vi "get_paths.vi"(8 "error in (no error)":errorcluster, 10 "force file name":string, 11 "GenericComponent in":refnum<class "GenericComponent.lvclass">) -> (0 "error out":errorcluster, 1 "settings paths":T3, 2 "configuration paths":T2, 3 "GenericComponent out":refnum<class "GenericComponent.lvclass">, 5 "component paths":T1)   [LabVIEW 2017, in "GenericComponent.lvclass"]
uses:
  GenericComponent.lvclass
  clusters/settings_paths_cluster.ctl
  clusters/configuration_paths_cluster.ctl
  component_path_clusters.ctl
  xcontrols/XUserDropdown/XUserDropdown/XUserDropdown.xctl
panel:
  # "(e.g., C:\\helioscan\\components\\Stage\\StageDL090602SutterMP285\\StageDL090602SutterMP285\\StageDL090602SutterMP285.lvclass)"
  # "(e.g., C:\\helioscan\\components\\Stage\\StageDL090602SutterMP285\\StageDL090602SutterMP285\\)"
  # "(e.g., C:\\helioscan\\components\\Stage)"
  # "(e.g., C:\\helioscan\\components)"
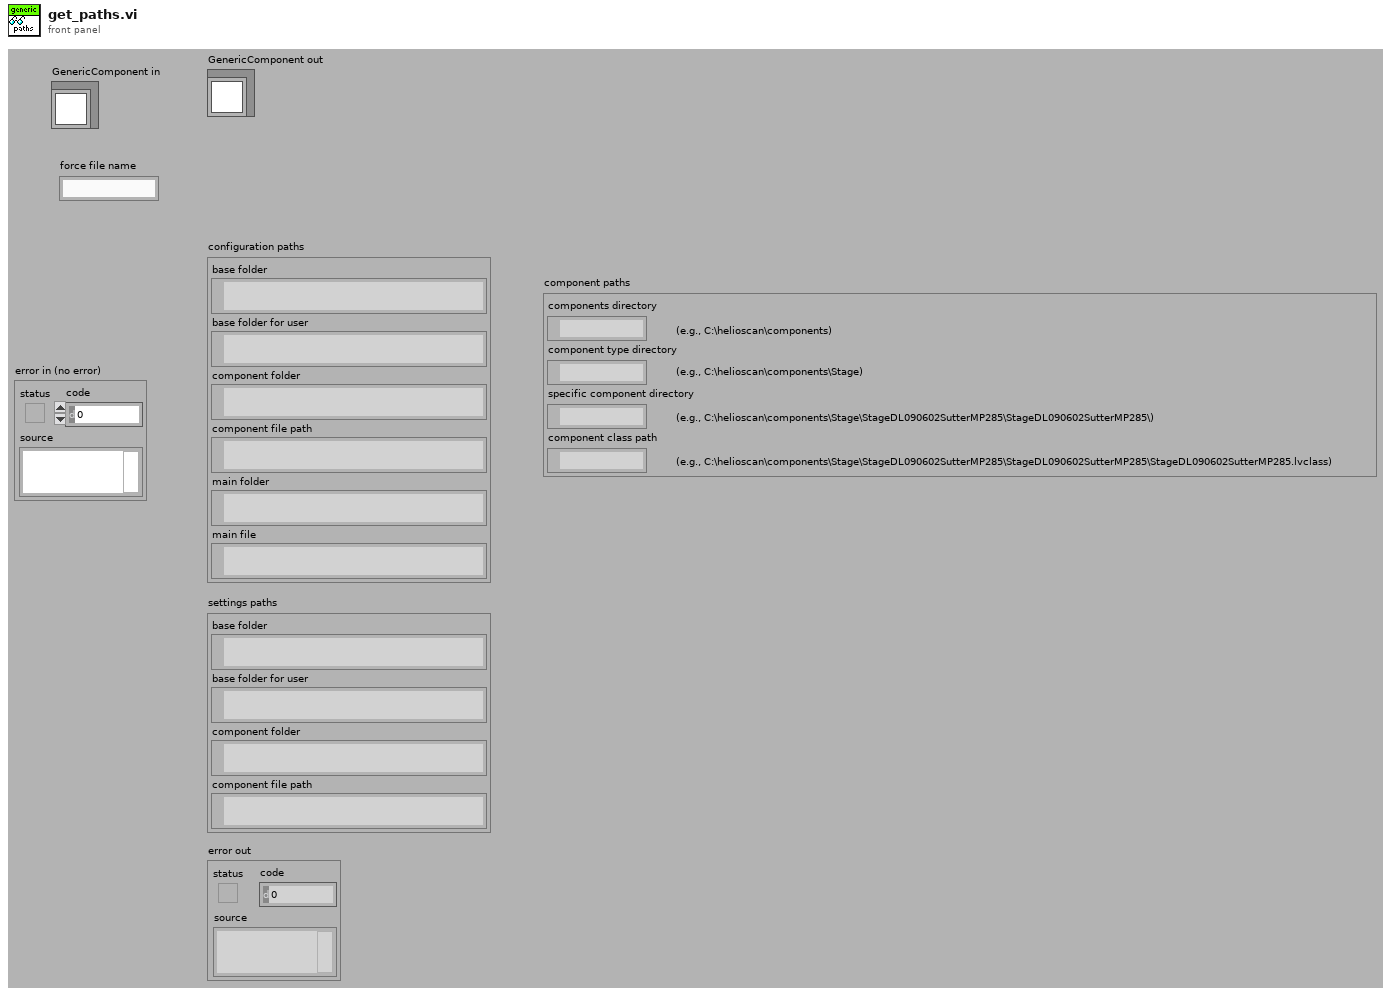
[diagram p1: front panel]
types:
  T1 = typedef "component_path_clusters.ctl" = cluster{"components directory":path, "component type directory":path, "specific component directory":path, "component class path":path}
  T2 = typedef "configuration_paths_cluster.ctl" = cluster{"base folder":path, "base folder for user":path, "component folder":path, "component file path":path, "main folder":path, "main file":path}
  T3 = typedef "settings_paths_cluster.ctl" = cluster{"base folder":path, "base folder for user":path, "component folder":path, "component file path":path}
  T4 = typedef "plugin_specification.ctl" = cluster{"class path":string, "configuration":string, "label":string, "settings name":string}
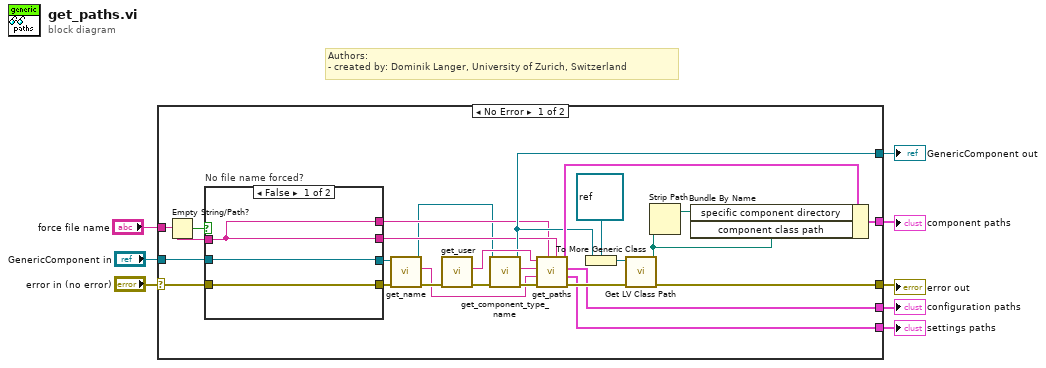
[diagram p0: block diagram]
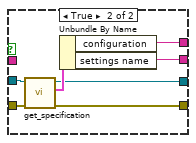
[diagram p2: hidden frame]
diagram:
  # "Authors: \n- created by: Dominik Langer, University of Zurich, Switzerland"
  n1 = case shown="No Error" "error in (no error)" {
    selector: "error in (no error)" -> [w16 w46]
    tunnel: [w13 w46] -> w4
    tunnel: [w20 _] -> w8
    tunnel: "GenericComponent in" -> [w17 w45]
    tunnel: [w19 _] -> w6
    tunnel: [w12 w45] -> w3
    tunnel: "force file name" -> [w18 _]
    tunnel: [w33 _] -> w1
    frame No Error {
      n2 = Empty String/Path?(string/path=w18) -> (empty?=w34:bool)
      n3 = case "No file name forced?" shown="False" w34 {
        tunnel: w16 -> [w36 w44]
        tunnel: [w36 w42] -> w14
        tunnel: w17 -> [w37 w43]
        tunnel: [w35 w39] -> w10
        tunnel: [w37 w38] -> w15
        tunnel: w18 -> [w35 _]
        tunnel: [w35 w40] -> w11
        frame False {
        }
        frame True {
          n4 = call-dynamic "get_specification.vi"("error in (no error)"=w44, "GenericPlugin in"=w43) -> ("error out"=w42:errorcluster, "component specification"=w41:T4, "GenericPlugin out"=w38:refnum<class "GenericComponent.lvclass">)  [unwired: 6 in, 1 out]
          n5 = Unbundle By Name(w41) -> ("configuration"=w39:string, "settings name"=w40:string)
        }
      }
      n6 = call-dynamic "get_name.vi"("error in (no error)"=w14, "GenericPlugin in"=w15) -> ("error out"=w22:errorcluster, "component name"=w21:string, "GenericPlugin out"=w9:refnum<class "GenericComponent.lvclass">)  [unwired: 7 in]
      n7 = call "get_user.vi"("error in (no error)"=w22) -> ("error out"=w24:errorcluster, "username out"=w25:string)  [unwired: 9 in]
      n8 = call-dynamic "get_component_type_name.vi"("error in (no error)"=w24, "GenericPlugin in"=w9) -> ("error out"=w27:errorcluster, "component type"=w26:string, "GenericPlugin out"=w12:refnum<class "GenericComponent.lvclass">)  [unwired: 7 in]
      n9 = call "get_paths.vi"("settings file name (without ending)"=w11, "configuration file name (without ending)"=w10, "error in (no error)"=w27, "component name"=w21, "component type"=w26, "user"=w25) -> ("error out"=w23:errorcluster, "settings paths"=w19:T3, "configuration paths"=w20:T2, "component paths"=w28:T1)  [unwired: 2 in]
      n10 = To More Generic Class(target class=refnum<class> refnum ("LabVIEW Object"), reference=w12) -> (generic class reference=w32:refnum<class>)
      n11 = call <vilib>:"Get LV Class Path.vi"("error in (no error)"=w23, "object"=w32) -> ("error out"=w13:errorcluster, "class path"=w29:path)  [unwired: 8 in]
      n12 = Strip Path(path=w29) -> (stripped path=w30:path)  [unwired: 1 out]
      n13 = Bundle By Name(cluster=w28, "specific component directory"=w30, "component class path"=w29) -> (w33:T1)
    }
    frame Error {
    }
  }
  "error out" <- w4
  "GenericComponent out" <- w3
  "settings paths" <- w6
  "configuration paths" <- w8
  "component paths" <- w1
